vi "FPGA Start FIFO.vi"(8 "error in (no error)":errorcluster, 10 "FIFO":T1, 11 "FPGA Session In":refnum<class "FPGA Interface By TypeDefs.lvclass">) -> (0 "error out":errorcluster, 3 "FPGA Session Out":refnum<class "FPGA Interface By TypeDefs.lvclass">)   [LabVIEW 2010, in "FPGA Interface By TypeDefs.lvclass"]
doc: "Starts a FIFO."
uses:
  FPGA Interface By TypeDefs.lvclass
  TypeDefs/AllFifos.ctl
  <userlib>/_FPGA Interface Advanced Tools/FPGA Interface Base/FPGA Interface Base.lvclass/FPGA Interface Base.ctl
  <vilib>/Utility/error.llb/Error Cluster From Error Code.vi
  <userlib>/_FPGA Interface Advanced Tools/FPGA Interface Base/Accessors/FPGA Read Session.vi
  <userlib>/_FPGA Interface Advanced Tools/FPGA Interface Wrapper/FPGA Interface Wrapper.lvlib
  <userlib>/_FPGA Interface Advanced Tools/FPGA Interface Base/FPGA Interface Base.lvclass
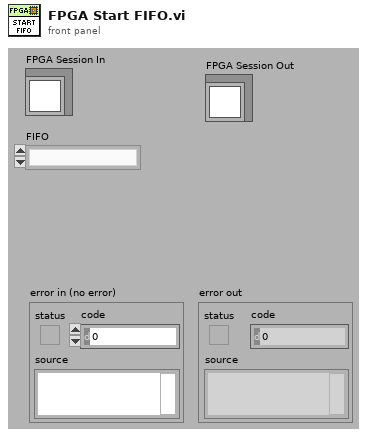
[diagram p1: front panel]
types:
  T1 = typedef "FPGA Interface By TypeDefs.lvclass/AllFifos.ctl" = enum16{""}
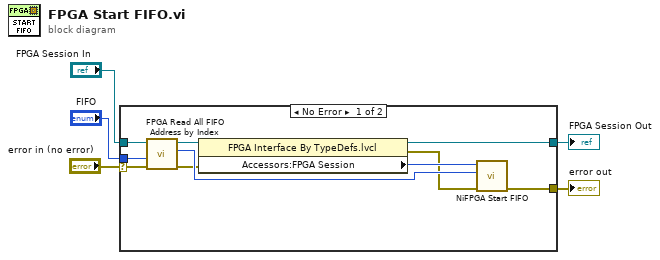
[diagram p0: block diagram]
diagram:
  n1 = case shown="No Error" "error in (no error)" {
    selector: "error in (no error)" -> [w14 w17]
    tunnel: [w7 w17] -> w2
    tunnel: [w8 w16] -> w1
    tunnel: "FPGA Session In" -> [w15 w16]
    tunnel: "FIFO" -> [w6 _]
    frame No Error {
      n2 = call <userlib>:"FPGA Read All FIFO Address by Index.vi"("error in (no error)"=w14, "index"=w6, "FPGA Interface Base in"=w15) -> ("error out"=w11:errorcluster, "Address"=w13:u32, "FPGA Interface Base out"=w12:refnum<class "FPGA Interface By TypeDefs.lvclass">)  [unwired: 5 in, 1 out]
      n3 = property class="FPGA Interface By TypeDefs.lvcl"(reference=w12, error in=w11) -> (reference out=w8:refnum<class "FPGA Interface By TypeDefs.lvclass">, error out=w9:errorcluster, "Accessors:FPGA Session"=w10:u32)
      n4 = call <userlib>:"NiFPGA Start FIFO.vi"("error in (no error)"=w9, "FIFO"=w13, "Session"=w10) -> ("error out"=w7:errorcluster)  [unwired: 7 in, 1 out]
    }
    frame Error {
    }
  }
  "error out" <- w2
  "FPGA Session Out" <- w1
